vi "Write JSON Config.vi"(6 "Pretty Print?":bool, 8 "error in (no error)":errorcluster, 11 "Subset_STR in":refnum<class "Subset_STR.lvclass">) -> (0 "error out":errorcluster, 2 "JSON":string, 3 "Subset_STR out":refnum<class "Subset_STR.lvclass">)   [LabVIEW 2021, in "Subset_STR.lvclass"]
uses:
  Subset_STR.lvclass
  Abs_Types/String/Abs_String.lvclass
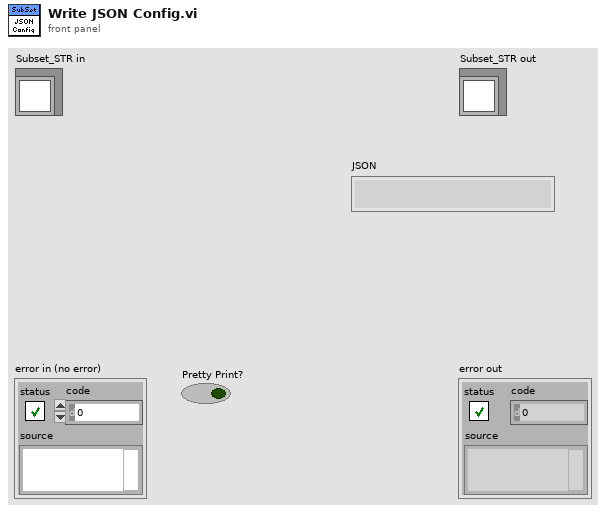
[diagram p1: front panel]
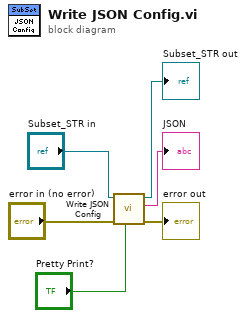
[diagram p0: block diagram]
diagram:
  n1 = call-parent "Write JSON Config.vi"("Pretty Print?"="Pretty Print?", "error in (no error)"="error in (no error)", "Abs_Type in"="Subset_STR in") -> ("error out"=→"error out":errorcluster, "JSON"=→"JSON":string, "Abs_Type out"=→"Subset_STR out":refnum<class "Subset_STR.lvclass">)  [unwired: 6 in]
